vi "LUT.grey-red.vi"() -> (0 "grey-red Palette":cluster{u8, u8, u8}[](array[cluster]))   [LabVIEW 2013]
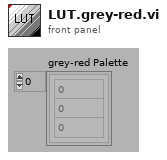
[diagram p1: front panel]
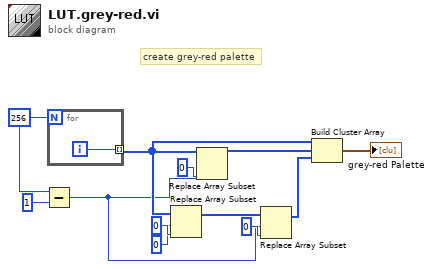
[diagram p0: block diagram]
diagram:
  w2 = 256
  # "create grey-red palette"
  n1 = Subtract(x=w2, y=u8 1) -> (x-y=w1:i32)
  n2 = for {
    N: w2 -> [_]
    tunnel: [w13] -> w9 mode=indexing
    i -> [w13]
  }
  n3 = Replace Array Subset(array=w9, new element=0, index=0) -> (w11:i32[])
  n4 = Replace Array Subset(array=w9, new element=0, index=w1) -> (w8:i32[])
  n5 = Replace Array Subset(array=w11, new element=0, index=w1) -> (w10:i32[])
  n6 = Build Cluster Array(w9, w8, w10) -> (→"grey-red Palette":cluster{i32, i32, i32}[])
